vi "Dummy VI 1.vi"() -> ()   [LabVIEW 2020]
panel:
  in  "file path (use dialog)":path
  out "Numeric out":i32
  in  "Numeric in":i32
  out "error out":errorcluster
  in  "error in":errorcluster
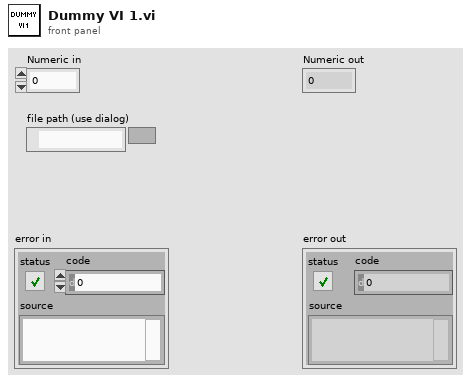
[diagram p1: front panel]
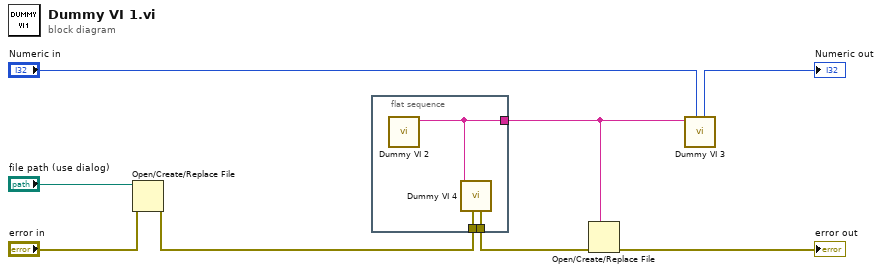
[diagram p0: block diagram]
diagram:
  n1 = Open/Create/Replace File(file path (use dialog)="file path (use dialog)", error in="error in") -> (error out=w5:errorcluster)  [unwired: 4 in, 2 out]
  n2 = flat-sequence {
    tunnel: w5 -> [w11]
    tunnel: [w10] -> w3
    tunnel: [w9] -> w2
    frame #0 {
      n3 = call "Dummy VI 2.vi"() -> ("String"=w9:string)  [unwired: 11 in]
      n4 = call "Dummy VI 4.vi"("error in"=w11, "String"=w9) -> ("error out"=w10:errorcluster)  [unwired: 9 in]
    }
  }
  n5 = Open/Create/Replace File(error in=w3, prompt=w2) -> (error out=→"error out":errorcluster)  [unwired: 4 in, 2 out]
  n6 = call "Dummy VI 3.vi"("Numeric in"="Numeric in", "String in"=w2) -> ("Numeric out"=→"Numeric out":i32)  [unwired: 8 in, 1 out]
